vi "Global.vi"() -> ()   [LabVIEW 2022 SP3, in "CSV Export.lvlib" / "CSV Export.lvclass"]
uses:
  CSV Export.lvclass
panel:
  in  "Attribute ID":string="CSV_Export_Alias"
  # "This is used to check the global attribute manager to ensure only a single instance of this plugin is used."
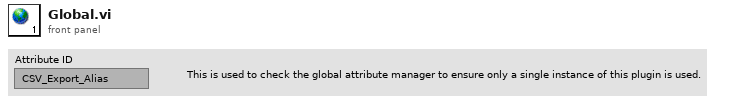
[diagram p1: front panel]
diagram:
